vi "Read Weighting.vi"(8 "error in (no error)":errorcluster, 11 "Noise in":refnum<class "Noise.lvclass">) -> (0 "error out":errorcluster, 2 "Weights":T1, 3 "Noise out":refnum<class "Noise.lvclass">)   [LabVIEW 2020, in "Noise.lvclass"]
uses:
  Noise.lvclass
  Weighting.ctl
  Noise.lvclass/Noise.ctl
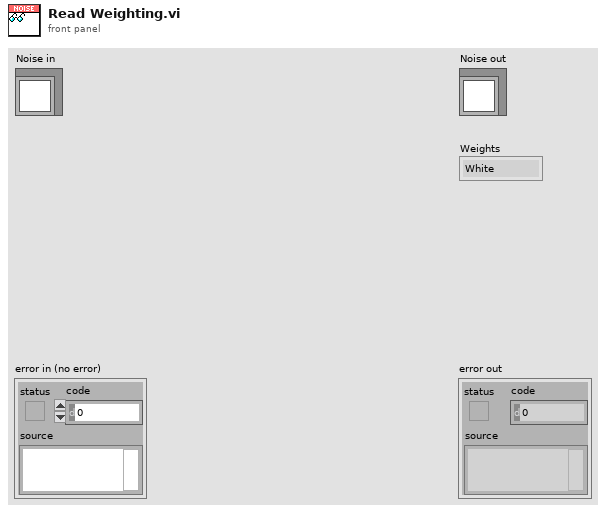
[diagram p1: front panel]
types:
  T1 = typedef "Noise.lvclass/Weighting.ctl" = enum16{"White", "Pink"}
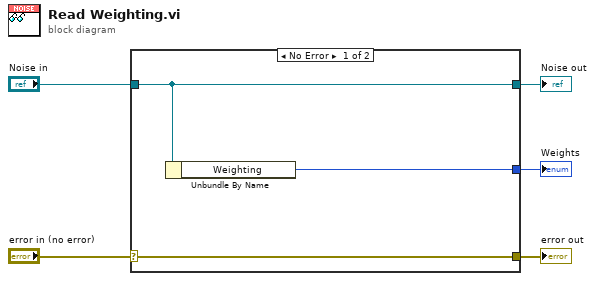
[diagram p0: block diagram]
diagram:
  n1 = case shown="No Error" "error in (no error)" {
    selector: "error in (no error)" -> [w8 w9]
    tunnel: [w8 w9] -> w4
    tunnel: [w7 w10] -> w2
    tunnel: "Noise in" -> [w7 w10]
    tunnel: [w6 _] -> w1
    frame No Error {
      n2 = Unbundle By Name(w7) -> ("Weighting"=w6:T1)
    }
    frame Error {
    }
  }
  "error out" <- w4
  "Noise out" <- w2
  "Weights" <- w1
